vi "sir_v1.vi"() -> ()   [LabVIEW 2009]
panel:
  in  "stop":bool
  out "Afisare sir de caractere":string="Aplicatie LabWIEW \n"
  in  "Introducere sir de caractere":string="Aplicatie LabWIEW \n"
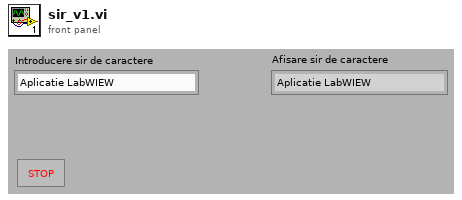
[diagram p1: front panel]
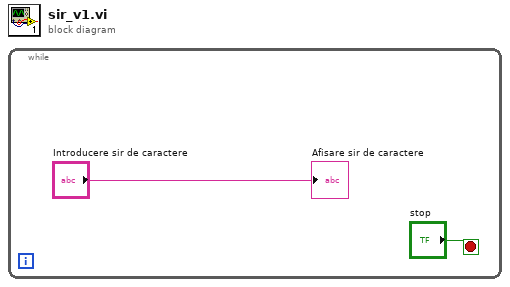
[diagram p0: block diagram]
diagram:
  n1 = while {
    stop <- "stop" stop-if-true
    "Afisare sir de caractere" <- "Introducere sir de caractere"
  }
